vi "NIIE_KeyDown.vi"(6 "PlatMods":T9, 7 "Type":T1, 8 "Error":errorcluster, 9 "VKey":T10, 10 "Char":i16, 11 "Data":T2={"Class"={"Ants"=refnum, "Layer"=refnum, "Templates"=refnum, "Icon"=refnum, "Glyph"=refnum, "Settings"=refnum, "Tools"=refnum}, "Ref"={"Add Layer"=refnum, "Remove Layer"=refnum, "Line Text"=[], "Body Text Spec"=refnum, "DNL_Font"=refnum, "glyph path str"=refnum, "templates path str"=refnum, "Arrow Up"=refnum, "Arrow Down"=refnum, "IE VI Ref"=refnum, "Glyphs tree"=refnum, "Templates tree"=refnum, "Layer Icon Text"=refnum, "Layer Template"=refnum, "Clipboard"=refnum, "BW icon in"=refnum, "Color icon in"=refnum, "Layer Clust"=refnum, "Body Text"=refnum, "DNL_Framework Templates"=refnum, "Search Templates"=refnum, "TextMarker"=refnum, "Tab Control"=refnum, "Search Glyphs"=refnum, "Line Color"=refnum, "DNL_Glyphs []"=refnum, "Fill Color"=refnum, "Tools"=refnum, "Glyphs tree"=refnum, "Icon"=refnum, "Preview"=refnum, "Ants"=refnum, "Terminals"=refnum, "menu reference"=refnum, "LayerNames"=[], "GlyphLoadAnimation"=refnum, "TemplateLoadAnimation"=refnum, "refreshGlyphs"=refnum, "refreshTemplates"=refnum}, "Support"={"AntsRect"={"left"=0, "top"=0, "right"=0, "bottom"=0}, "Mouse Move Coords"={"Horizontal"=0, "Vertical"=0}, "Mouse Down Coords"={"Horizontal"=0, "Vertical"=0}, "Temp Coord"={"Horizontal"=0, "Vertical"=0}, "Action"=enum."Default", "Edge Color"=4914962, "Fill Color"=16860, "Mouse Down?"=FALSE, "Draft Mode?"=FALSE, "Temp Icon"=bytes[3102], "CTRL Pressed"=FALSE, "Move Selection?"=FALSE, "AntsRect Orig"={"left"=0, "top"=0, "right"=0, "bottom"=0}, "Text"="", "TM Set?"=FALSE, "Mouse inside icon?"=FALSE, "Tool (old value)"=0, "Pencil Move Color"=0, "Swap Colors?"=FALSE, "Shift pressed?"=FALSE}}) -> (0 "Error Out":errorcluster, 1 "Discard? Out":bool, 3 "Data Out":T2={"Class"={"Ants"=refnum, "Layer"=refnum, "Templates"=refnum, "Icon"=refnum, "Glyph"=refnum, "Settings"=refnum, "Tools"=refnum}, "Ref"={"Add Layer"=refnum, "Remove Layer"=refnum, "Line Text"=[], "Body Text Spec"=refnum, "DNL_Font"=refnum, "glyph path str"=refnum, "templates path str"=refnum, "Arrow Up"=refnum, "Arrow Down"=refnum, "IE VI Ref"=refnum, "Glyphs tree"=refnum, "Templates tree"=refnum, "Layer Icon Text"=refnum, "Layer Template"=refnum, "Clipboard"=refnum, "BW icon in"=refnum, "Color icon in"=refnum, "Layer Clust"=refnum, "Body Text"=refnum, "DNL_Framework Templates"=refnum, "Search Templates"=refnum, "TextMarker"=refnum, "Tab Control"=refnum, "Search Glyphs"=refnum, "Line Color"=refnum, "DNL_Glyphs []"=refnum, "Fill Color"=refnum, "Tools"=refnum, "Glyphs tree"=refnum, "Icon"=refnum, "Preview"=refnum, "Ants"=refnum, "Terminals"=refnum, "menu reference"=refnum, "LayerNames"=[], "GlyphLoadAnimation"=refnum, "TemplateLoadAnimation"=refnum, "refreshGlyphs"=refnum, "refreshTemplates"=refnum}, "Support"={"AntsRect"={"left"=0, "top"=0, "right"=0, "bottom"=0}, "Mouse Move Coords"={"Horizontal"=0, "Vertical"=0}, "Mouse Down Coords"={"Horizontal"=0, "Vertical"=0}, "Temp Coord"={"Horizontal"=0, "Vertical"=0}, "Action"=enum."Default", "Edge Color"=4914962, "Fill Color"=16860, "Mouse Down?"=FALSE, "Draft Mode?"=FALSE, "Temp Icon"=bytes[3102], "CTRL Pressed"=FALSE, "Move Selection?"=FALSE, "AntsRect Orig"={"left"=0, "top"=0, "right"=0, "bottom"=0}, "Text"="", "TM Set?"=FALSE, "Mouse inside icon?"=FALSE, "Tool (old value)"=0, "Pencil Move Color"=0, "Swap Colors?"=FALSE, "Shift pressed?"=FALSE}})   [LabVIEW 2021]
uses:
  <vilib>/event_ctls.llb/eventvkey.ctl
  Controls/IE Data.ctl
  Class/Ants/Ants.lvclass
  Class/FakedArray/FakedArray.lvclass
  Class/Icon Library/Glyph.lvclass
  Class/Settings/Settings.lvclass
  Class/Tools/Tools Paint.lvclass
  vi.lib/LabVIEW Icon API/lv_icon/Classes/Icon/Icon.lvclass
  Controls/IE Classes.ctl
  Controls/References Cluster.ctl
  Controls/SupportClass.ctl
  <vilib>/Utility/miscctls.llb/LVPoint32TypeDef.ctl
  Controls/ENUM_SupportClass_Action.ctl
  vi.lib/LabVIEW Icon API/lv_icon/Controls/IEColor.ctl
  <vilib>/event_ctls.llb/lveventtype.ctl
  vi.lib/LabVIEW Icon API/lv_icon/lv_icon.lvlib
panel:
  in  "Layer name":string="Clipboard"
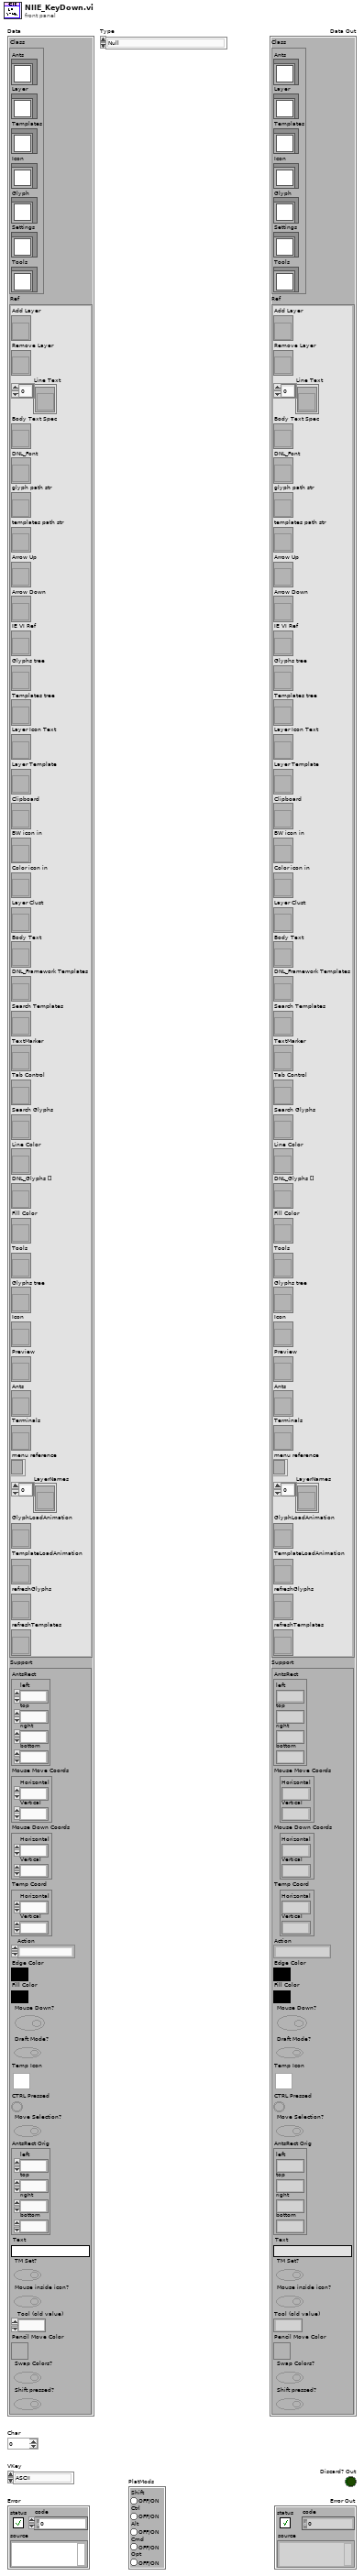
[diagram p1: front panel]
types:
  T1 = typedef "lveventtype.ctl" = enum32{"Null", "Timeout", "Annotation Menu Selection", "Annotation Menu Selection?", "App Instance Close", "App Instance Close?", "Autoscale Range Change", "Bookmark Info Change", "Cell Edit", "Cell Edit?", "Cursor Grab", "Cursor Grab?", "Cursor Menu Selection", "Cursor Menu Selection?", "Cursor Move", "Cursor Release", "Data Change", "Direction Change", "Display State Change", "Drag Ended", "Drag Enter", "Drag Leave", "Drag Over", "Drag Source Update", "Drag Starting", "Drag Starting?", "Drop", "Exec State Change", "Key Down", "Key Down?", "Key Repeat", "Key Repeat?", "Key Up", "Listbox Double Click", "Menu Activation?", "Menu Selection (App)", "Menu Selection? (App)", "Menu Selection (User)", "Mouse Down", "Mouse Down?", "Mouse Enter", "Mouse Leave", "Mouse Move", "Mouse Up", "Mouse Wheel", "NI Security User Change (App)", "Pane Size", "Panel Close", "Panel Close?", "Panel Resize", "Plot Attribute Change", "Scale Range Change", "Shortcut Menu Activation?", "Shortcut Menu Selection (App)", "Shortcut Menu Selection? (App)", "Shortcut Menu Selection (User)", "Tree Double Click", "Tree Drag", "Tree Drag?", "Tree Drop", "Tree Drop?", "Tree Item Close", "Tree Item Close?", "Tree Item Open", "Tree Item Open?", "User Event", "Value Change"}
  T2 = typedef "IE Data.ctl" = cluster{"Class":T3, "Ref":T4, "Support":T5}
  T3 = typedef "IE Classes.ctl" = cluster{"Ants":refnum<class "Ants.lvclass">, "Layer":refnum<class "FakedArray.lvclass">, "Templates":refnum<class "FakedArray.lvclass">, "Icon":refnum<class "Icon.lvclass">, "Glyph":refnum<class "Glyph.lvclass">, "Settings":refnum<class "Settings.lvclass">, "Tools":refnum<class "Tools Paint.lvclass">}
  T4 = typedef "References Cluster.ctl" = cluster{"Add Layer":refnum<vi>, "Remove Layer":refnum<vi>, "Line Text":refnum<vi>[], "Body Text Spec":refnum<vi>, "DNL_Font":refnum<vi>, "glyph path str":refnum<vi>, "templates path str":refnum<vi>, "Arrow Up":refnum<vi>, "Arrow Down":refnum<vi>, "IE VI Ref":refnum<vi>, "Glyphs tree":refnum<vi>, "Templates tree":refnum<vi>, "Layer Icon Text":refnum<vi>, "Layer Template":refnum<vi>, "Clipboard":refnum<vi>, "BW icon in":refnum<vi>, "Color icon in":refnum<vi>, "Layer Clust":refnum<vi>, "Body Text":refnum<vi>, "DNL_Framework Templates":refnum<vi>, "Search Templates":refnum<vi>, "TextMarker":refnum<vi>, "Tab Control":refnum<vi>, "Search Glyphs":refnum<vi>, "Line Color":refnum<vi>, "DNL_Glyphs []":refnum<vi>, "Fill Color":refnum<vi>, "Tools":refnum<vi>, "Glyphs tree":refnum<vi>, "Icon":refnum<vi>, "Preview":refnum<vi>, "Ants":refnum<vi>, "Terminals":refnum<vi>, "menu reference":refnum<k9>, "LayerNames":refnum<vi>[], "GlyphLoadAnimation":refnum<vi>, "TemplateLoadAnimation":refnum<vi>, "refreshGlyphs":refnum<vi>, "refreshTemplates":refnum<vi>}
  T5 = typedef "SupportClass.ctl" = cluster{"AntsRect":cluster{"left":i16, "top":i16, "right":i16, "bottom":i16}, "Mouse Move Coords":T6, "Mouse Down Coords":T6, "Temp Coord":T6, "Action":T7, "Edge Color":T8, "Fill Color":T8, "Mouse Down?":bool, "Draft Mode?":bool, "Temp Icon":picture, "CTRL Pressed":bool, "Move Selection?":bool, "AntsRect Orig":cluster{"left":i16, "top":i16, "right":i16, "bottom":i16}, "Text":string, "TM Set?":bool, "Mouse inside icon?":bool, "Tool (old value)":u32, "Pencil Move Color":u32, "Swap Colors?":bool, "Shift pressed?":bool}
  T6 = typedef "LVPoint32TypeDef.ctl" = cluster{"Horizontal":i32, "Vertical":i32}
  T7 = typedef "ENUM_SupportClass_Action.ctl" = enum16{"Default", "Move Selection", "Glyph Library", "Tool"}
  T8 = typedef "IEColor.ctl" = u32
  T9 = cluster{"Shift":bool, "Ctrl":bool, "Alt":bool, "Cmd":bool, "Opt":bool}
  T10 = typedef "eventvkey.ctl" = enum16{"ASCII", "Enter", "Return", "Shift", "Ctrl", "Alt", "Cmd", "Opt", "Caps", "NumLock", "Clear", "Break", "Up", "Down", "Left", "Right", "Insert", "Delete", "Home", "End", "PageUp", "PageDown", "Escape", "Help", "Pause", "ScrollLock", "F1", "F2", "F3", "F4", "F5", "F6", "F7", "F8", "F9", "F10", "F11", "F12", "F13", "F14", "F15", "F16", "F17", "F18", "F19", "F20", "F21", "F22", "F23", "F24", "Play", "VolumeUp", "VolumeDown", "Mute", "Two Byte Char"}
  T11 = cluster{"left":i16, "top":i16, "right":i16, "bottom":i16}
  T12 = enum32{"Pencil", "Line", "Dropper", "Fill", "Rectangle", "Filled Rectangle", "Ellipse", "Filled Ellipse", "Eraser", "Text", "Select", "Move"}
  T13 = typedef "Cluster_Path&Icon.ctl" = cluster{"Rectangle":cluster{"left":i16, "top":i16, "right":i16, "bottom":i16}, "Path":path, "Image":picture, "Filter":string, "FileName":string}
  T14 = cluster{"left":i16, "top":i16, "bottom":i16, "right":i16}
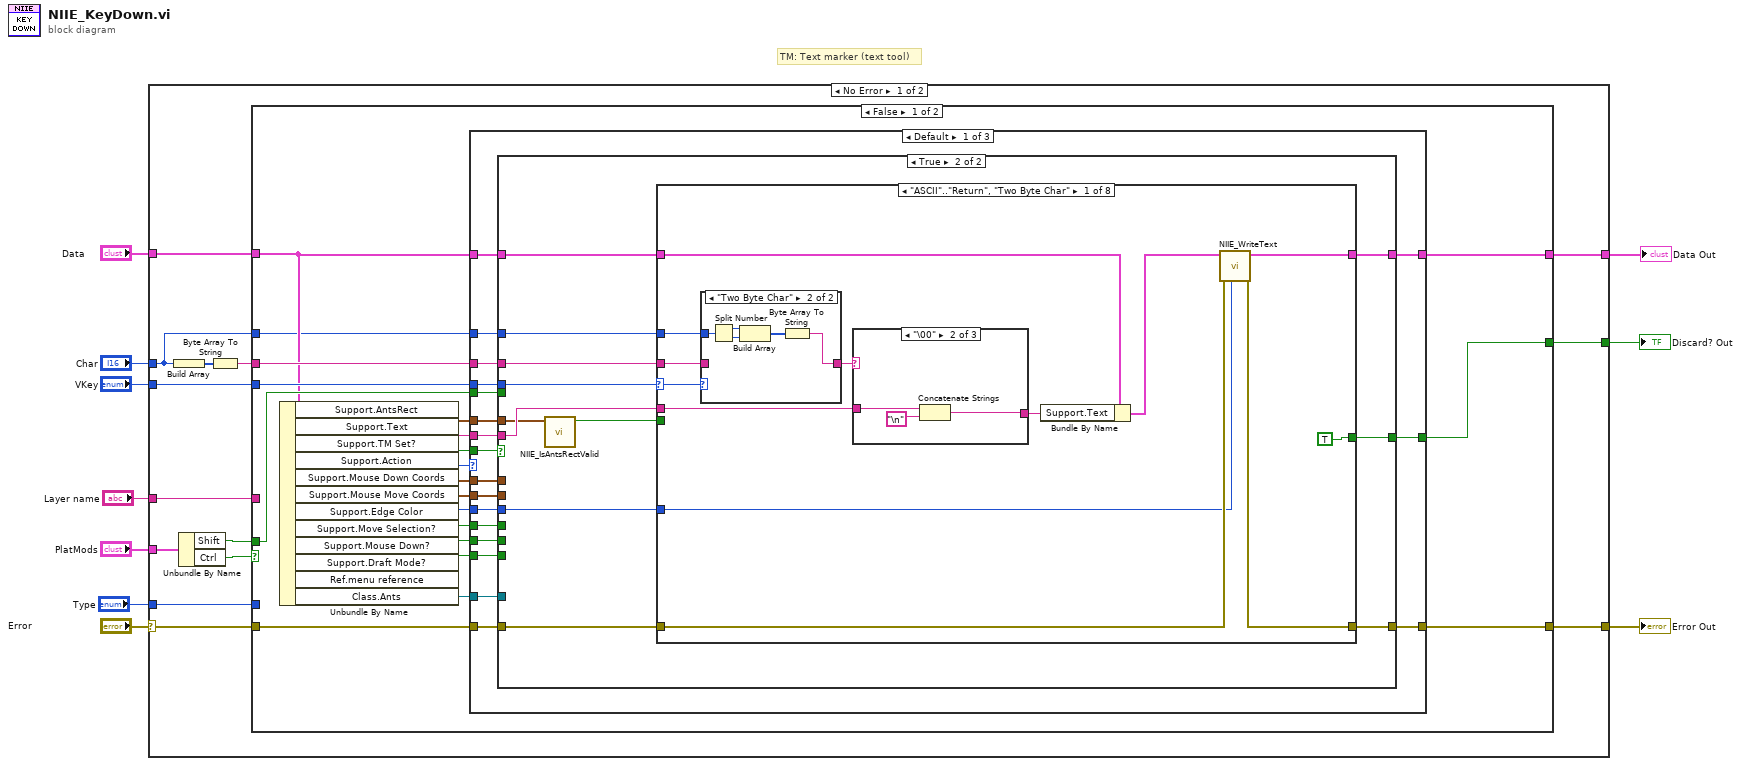
[diagram p0: block diagram]
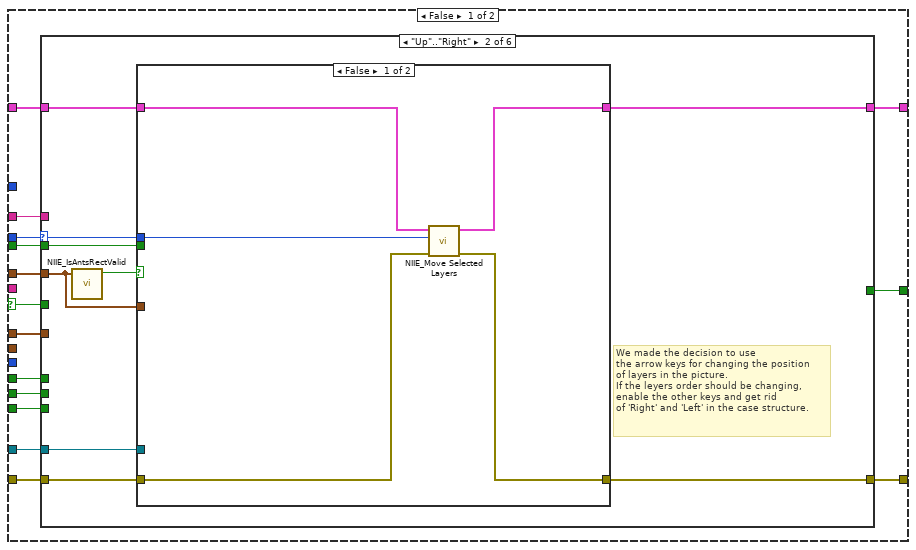
[diagram p2: hidden frame]
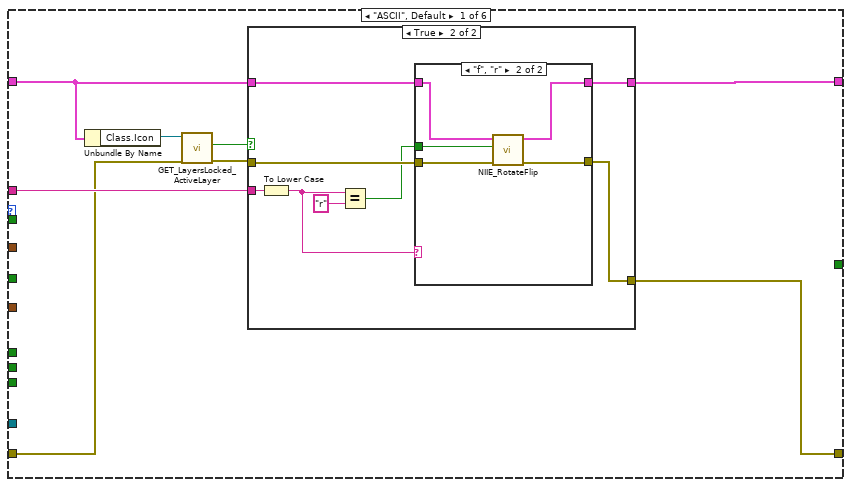
[diagram p3: hidden frame]
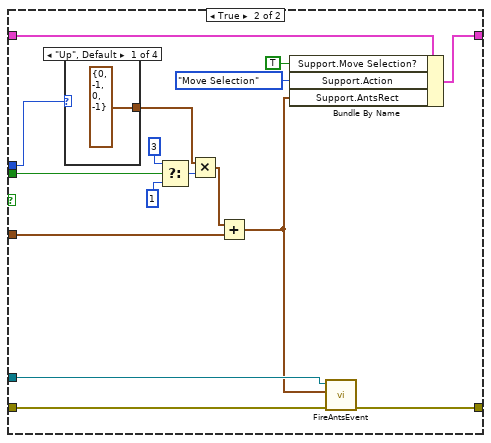
[diagram p6: hidden frame]
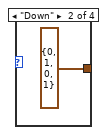
[diagram p7: hidden frame]
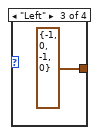
[diagram p8: hidden frame]
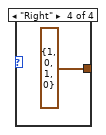
[diagram p9: hidden frame]
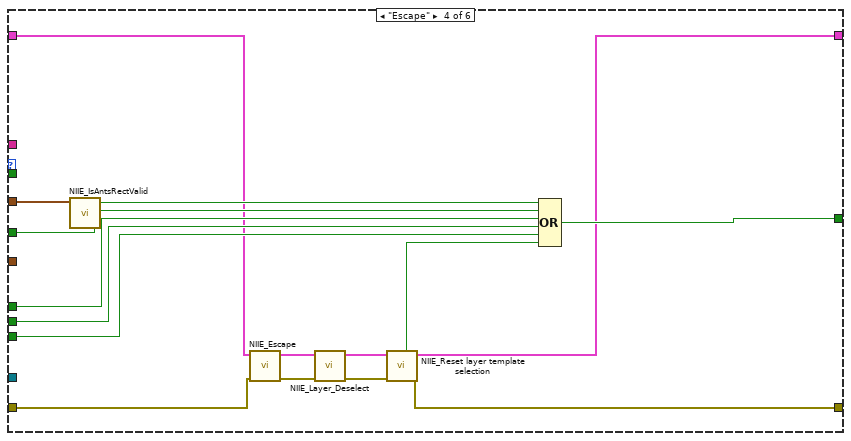
[diagram p11: hidden frame]
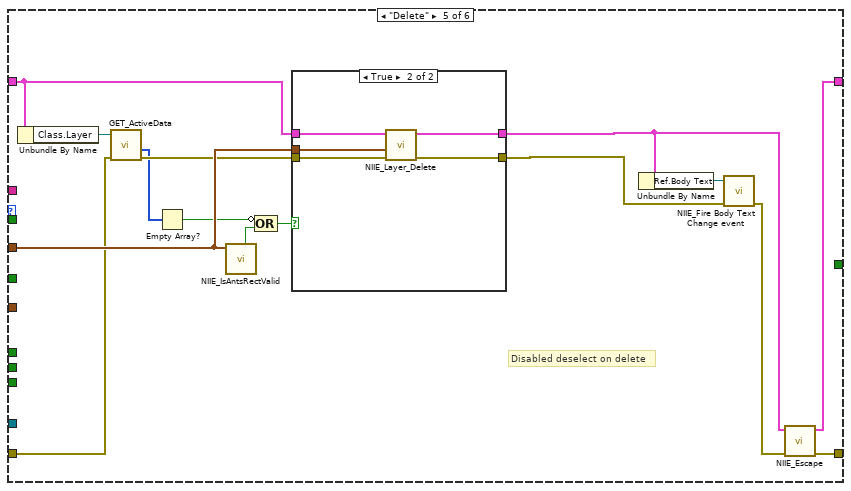
[diagram p12: hidden frame]
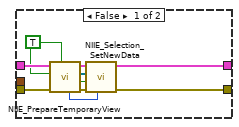
[diagram p13: hidden frame]
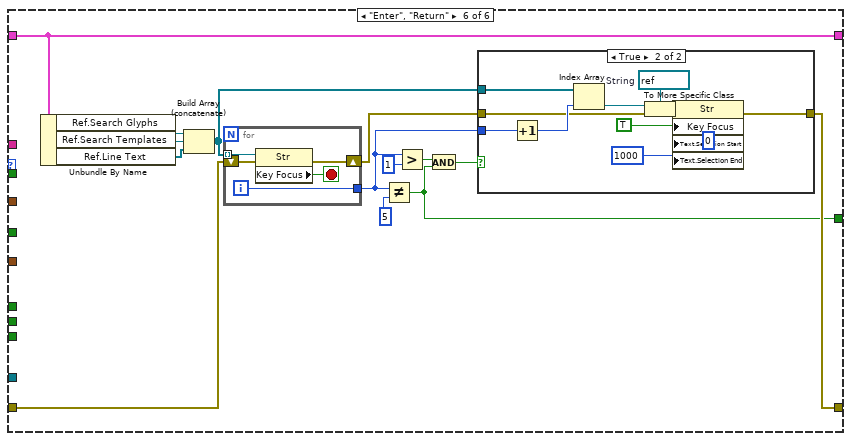
[diagram p14: hidden frame]
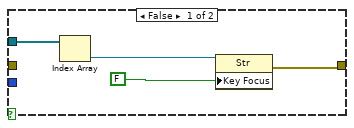
[diagram p15: hidden frame]
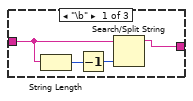
[diagram p17: hidden frame]
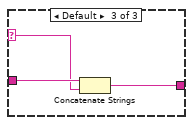
[diagram p18: hidden frame]
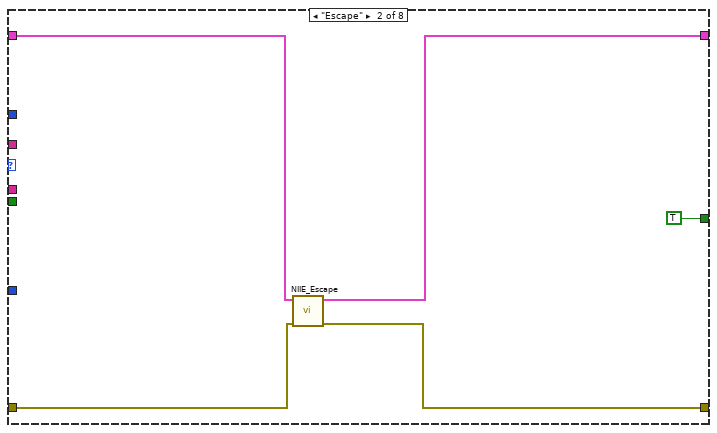
[diagram p19: hidden frame]
diagram:
  # "TM: Text marker (text tool)"
  n1 = case shown="No Error" "Error" {
    selector: "Error" -> [w17 w697]
    tunnel: [w21 w697] -> w9
    tunnel: "VKey" -> [w24 _]
    tunnel: "Char" -> [w12 _]
    tunnel: "PlatMods" -> [w20 _]
    tunnel: [w18 _] -> w5
    tunnel: "Data" -> [w15 w696]
    tunnel: [w14 w696] -> w3
    tunnel: "Type" -> [w13 _]
    tunnel: "Layer name" -> [w11 _]
    frame No Error {
      n2 = Build Array(w12) -> (w23:i16[])
      n3 = Unbundle By Name(w20) -> ("Shift"=w16:bool, "Ctrl"=w19:bool)
      n4 = Byte Array To String(unsigned byte array=w23) -> (string=w22:string)
      n5 = case shown="False" w19 {
        selector: w19 -> [_ w484]
        tunnel: w24 -> [w44 _]
        tunnel: w22 -> [w43 w482]
        tunnel: [w28 w494] -> w21
        tunnel: [w32 w481] -> w18
        tunnel: w17 -> [w30 w497]
        tunnel: w16 -> [w31 w485]
        tunnel: w15 -> [w29 w496]
        tunnel: [w26 w495] -> w14
        tunnel: w13 -> [_ w489]
        tunnel: w12 -> [w25 _]
        tunnel: w11 -> [_ w479]
        frame False {
          n6 = Unbundle By Name(w29) -> ("Support.AntsRect"=w37:T11, "Support.Text"=w40:string, "Support.TM Set?"=w41:bool, "Support.Action"=w42:T7, "Support.Mouse Down Coords"=w39:T6, "Support.Mouse Move Coords"=w36:T6, "Support.Edge Color"=w38:T8, "Support.Move Selection?"=w35:bool, "Support.Mouse Down?"=w34:bool, "Support.Draft Mode?"=w33:bool, "Class.Ants"=w27:refnum<class "Ants.lvclass">)  [unwired: 1 out]
          n7 = case shown="Default" w42 {
            tunnel: w44 -> [w63 w329 w396]
            tunnel: w43 -> [w58 w328 _]
            tunnel: w30 -> [w61 w327 w398]
            tunnel: [w62 w326 w397] -> w28
            tunnel: w41 -> [w60 w324 w394]
            tunnel: w40 -> [w59 _ _]
            tunnel: w39 -> [w57 _ _]
            tunnel: w38 -> [w56 _ _]
            tunnel: w37 -> [w55 w325 w395]
            tunnel: w36 -> [w54 w317 _]
            tunnel: w35 -> [w53 w323 w393]
            tunnel: w34 -> [w52 w322 w392]
            tunnel: w33 -> [w51 w321 w391]
            tunnel: [w50 w320 w390] -> w32
            tunnel: w31 -> [w49 _ w386]
            tunnel: w29 -> [w48 w319 w389]
            tunnel: [w47 w318 w388] -> w26
            tunnel: w27 -> [w45 _ w387]
            tunnel: w25 -> [w46 _ _]
            frame Default {
              n8 = case shown="True" w60 {
                selector: w60 -> [w69 _]
                tunnel: w63 -> [w77 w231]
                tunnel: [w76 w230] -> w62
                tunnel: w61 -> [w78 w229]
                tunnel: w59 -> [_ w228]
                tunnel: w58 -> [w75 w227]
                tunnel: w57 -> [w73 _]
                tunnel: w56 -> [_ w224]
                tunnel: w55 -> [w74 w226]
                tunnel: w54 -> [_ _]
                tunnel: w53 -> [w72 _]
                tunnel: w52 -> [w71 _]
                tunnel: w51 -> [w70 _]
                tunnel: [w68 w223] -> w50
                tunnel: w49 -> [w67 _]
                tunnel: w48 -> [w66 w222]
                tunnel: [w65 w221] -> w47
                tunnel: w46 -> [_ w220]
                tunnel: w45 -> [w64 _]
                frame False {
                  n9 = case shown="\"Up\"..\"Right\"" w77 {
                    selector: w77 -> [_ w110 _ _ _ _]
                    tunnel: w78 -> [w82 w112 w139 w155 w163 w198]
                    tunnel: [w85 w111 w139 w152 w170 w195] -> w76
                    tunnel: w75 -> [w86 _ _ _ _ _]
                    tunnel: w74 -> [_ w105 _ w150 w167 _]
                    tunnel: w73 -> [_ _ _ _ _ _]
                    tunnel: w72 -> [_ _ _ w148 _ _]
                    tunnel: w71 -> [_ _ _ w147 _ _]
                    tunnel: w70 -> [_ _ _ w146 _ _]
                    tunnel: w69 -> [_ _ _ w149 _ _]
                    tunnel: [_ _ _ w145 _ w187] -> w68
                    tunnel: w67 -> [_ w109 _ _ _ _]
                    tunnel: w66 -> [w84 w108 w138 w143 w164 w199]
                    tunnel: [w83 w107 w138 w140 w169 w199] -> w65
                    tunnel: w64 -> [_ w104 _ _ _ _]
                    frame "ASCII", Default {
                      n10 = Unbundle By Name(w84) -> ("Class.Icon"=w80:refnum<class "Icon.lvclass">)
                      n11 = call-dynamic "GET_LayersLocked_ActiveLayer.vi"("error in (no error)"=w82, "Icon.lvclass in"=w80) -> ("error out"=w81:errorcluster, "Layers Locked?"=w79:bool)  [unwired: 8 out]
                      n12 = case shown="True" w79 {
                        tunnel: w86 -> [_ w93]
                        tunnel: w81 -> [w88 w96]
                        tunnel: [w88 w95] -> w85
                        tunnel: w84 -> [w87 w90]
                        tunnel: [w87 w89] -> w83
                        frame False {
                        }
                        frame True {
                          n13 = To Lower Case(string=w93) -> (all lower case string=w91:string)
                          n14 = Equal?(x=w91, y="r") -> (x = y?=w92:bool)
                          n15 = case shown="\"f\", \"r\"" w91 {
                            tunnel: w96 -> [w98 w103]
                            tunnel: [w98 w101] -> w95
                            tunnel: w92 -> [_ w102]
                            tunnel: w90 -> [w97 w100]
                            tunnel: [w97 w99] -> w89
                            frame Default {
                            }
                            frame "f", "r" {
                              n16 = call "NIIE_RotateFlip.vi"("Error"=w103, "Rotate"=w102, "Data"=w100) -> ("Error Out"=w101:errorcluster, "Data Out"=w99:T2)  [unwired: 3 in, 4 out]
                            }
                          }
                        }
                      }
                    }
                    frame "Up".."Right" {
                      # "We made the decision to use\nthe arrow keys for changing the position\nof layers in the picture.\nIf the leyers order should be changing,\nenable the other keys and get rid\nof 'Right' and 'Left' in the case structure."
                      n17 = call "NIIE_IsAntsRectValid.vi"("Image Range"=w105) -> ("Valid? Out"=w106:bool)  [unwired: 10 out]
                      n18 = case shown="False" w106 {
                        tunnel: w112 -> [w117 w121]
                        tunnel: [w116 w120] -> w111
                        tunnel: w110 -> [w115 w124]
                        tunnel: w109 -> [_ w123]
                        tunnel: w108 -> [w114 w133]
                        tunnel: [w113 w131] -> w107
                        tunnel: w105 -> [_ w122]
                        tunnel: w104 -> [_ w119]
                        frame False {
                          n19 = call "NIIE_Move Selected Layers.vi"("Error"=w117, "VKey"=w115, "Data"=w114) -> ("Error Out"=w116:errorcluster, "Data Out"=w113:T2)  [unwired: 1 in, 6 out]
                        }
                        frame True {
                          n20 = case shown="\"Up\", Default" w124 {
                            tunnel: [T11 {"left"=0, "top"=-1, "right"=0, "bottom"=-1} ("y") T11 {"left"=0, "top"=1, "right"=0, "bottom"=1} ("y") T11 {"left"=-1, "top"=0, "right"=-1, "bottom"=0} ("y") T11 {"left"=1, "top"=0, "right"=1, "bottom"=0} ("y")] -> w129
                            frame "Up", Default {
                            }
                            frame "Down" {
                            }
                            frame "Left" {
                            }
                            frame "Right" {
                            }
                          }
                          n21 = Select(t=i16 3 ("left"), s=w123, f=i16 1 ("left")) -> (s? t:f=w126:i16)
                          n22 = Multiply(x=w129, y=w126) -> (x*y=w125:T11)
                          n23 = Add(x=w125, y=w122) -> (x+y=w118:T11)
                          n24 = Bundle By Name(cluster=w133, "Support.Move Selection?"=TRUE, "Support.Action"=ENUM_SupportClass_Action."Move Selection", "Support.AntsRect"=w118) -> (w131:T2)
                          n25 = call "FireAntsEvent.vi"("error in (no error)"=w121, "Rectangle (default: deselect)"=w118, "Ants in"=w119) -> ("error out"=w120:errorcluster)  [unwired: 1 in, 7 out]
                        }
                      }
                    }
                    frame "Shift" {
                    }
                    frame "Escape" {
                      n26 = call "NIIE_IsAntsRectValid.vi"("Image Range"=w150) -> ("Valid? Out"=w151:bool)  [unwired: 10 out]
                      n27 = call "NIIE_Escape.vi"("Error"=w155, "Data"=w143) -> ("Error Out"=w154:errorcluster, "Data Out"=w142:T2)  [unwired: 8 out]
                      n28 = call "NIIE_Layer_Deselect.vi"("Error"=w154, "Data"=w142) -> ("Error Out"=w153:errorcluster, "Data Out"=w141:T2)  [unwired: 8 out]
                      n29 = call "NIIE_Reset layer template selection.vi"("Error"=w153, "Data"=w141) -> ("Error Out"=w152:errorcluster, "Data Out"=w140:T2, "Layers Selected? Out"=w144:bool)  [unwired: 1 in, 6 out]
                      n30 = Compound Arithmetic op=OR(w151, w149, w148, w147, w146, w144) -> (w145:bool)
                    }
                    frame "Delete" {
                      # "Disabled deselect on delete"
                      n31 = Unbundle By Name(w164) -> ("Class.Layer"=w165:refnum<class "FakedArray.lvclass">)
                      n32 = call-dynamic "GET_ActiveData.vi"("Error"=w163, "FakedArray"=w165) -> ("Error Out"=w162:errorcluster, "Active Data [] Out"=w161:i32[])  [unwired: 4 in, 4 out]
                      n33 = Empty Array?(array=w161) -> (empty?=w159:bool)
                      n34 = call "NIIE_IsAntsRectValid.vi"("Image Range"=w167) -> ("Max. Rect Size? Out"=w160:bool)  [unwired: 10 out]
                      n35 = Compound Arithmetic op=OR(invert w159, w160) -> (w158:bool)
                      n36 = case shown="True" w158 {
                        tunnel: w164 -> [w180 w185]
                        tunnel: [w179 w183] -> w168
                        tunnel: [w178 w184] -> w157
                        tunnel: w162 -> [w171 w182]
                        tunnel: w167 -> [_ w181]
                        frame False {
                          w177 = TRUE ("Delete Selected Area?")
                          n37 = call "NIIE_PrepareTemporaryView.vi"("Delete Selected Area?"=w177, "Error"=w171, "Valid Selection?"=w177, "Data"=w180) -> ("Error Out"=w174:errorcluster, "Highlighted? Out"=w175:bool, "All Layers Out"=w176:refnum<class "Layer.lvclass">[], "Data Out"=w172:T2, "#Active Layer Out"=w173:i32)  [unwired: 1 in, 2 out]
                          n38 = call "NIIE_Selection_SetNewData.vi"("#Active Layer"=w173, "Error"=w174, "Highlighted?"=w175, "All Layers"=w176, "Data"=w172) -> ("Error Out"=w179:errorcluster, "Data Out"=w178:T2)  [unwired: 1 in, 3 out]
                        }
                        frame True {
                          n39 = call "NIIE_Layer_Delete.vi"("Error"=w182, "AntsRect"=w181, "Data"=w185) -> ("Error Out"=w183:errorcluster, "Data Out"=w184:T2)  [unwired: 5 out]
                        }
                      }
                      n40 = Unbundle By Name(w157) -> ("Ref.Body Text"=w156:refnum<vi>)
                      n41 = call "NIIE_Fire Body Text Change event.vi"("error in"=w168, "Ref.Body Text"=w156) -> ("error out"=w166:errorcluster)  [unwired: 2 in, 7 out]
                      n42 = call "NIIE_Escape.vi"("Error"=w166, "Data"=w157) -> ("Error Out"=w170:errorcluster, "Data Out"=w169:T2)  [unwired: 8 out]
                    }
                    frame "Enter", "Return" {
                      n43 = Unbundle By Name(w199) -> ("Ref.Search Glyphs"=w191:refnum<vi>, "Ref.Search Templates"=w192:refnum<vi>, "Ref.Line Text"=w194:refnum<vi>[])
                      n44 = Build Array (concatenate)(w191, w192, w194) -> (w193:refnum<vi>[])
                      n45 = for {
                        tunnel: w193 -> [w219] mode=indexing
                        shift-right: [w218] -> w196
                        shift-left: w198 -> [w217]
                        tunnel: [w216] -> w190
                        i -> [w216]
                        stop <- w215 stop-if-true
                        n46 = property class="Str"(reference=w219, error in=w217) -> (error out=w218:errorcluster, "Key Focus"=w215:bool)  [unwired: 1 out]
                      }
                      n47 = Not Equal?(x=w190, y=5) -> (x != y?=w187:bool)
                      n48 = Greater?(x=w190, y=1) -> (0:w188:bool)
                      n49 = And(x=w188, y=w187) -> (x .and. y?=w186:bool)
                      n50 = case shown="True" w186 {
                        tunnel: w190 -> [_ w213]
                        tunnel: w193 -> [w203 w214]
                        tunnel: w196 -> [_ w210]
                        tunnel: [w200 w208] -> w195
                        frame False {
                          n51 = Index Array(array=w203) -> (element=w202:refnum<vi>)  [unwired: 1 in]
                          n52 = property class="Str"(reference=w202, "Key Focus"=FALSE) -> (error out=w200:errorcluster)  [unwired: 1 in, 1 out]
                        }
                        frame True {
                          w204 = refnum<vi> refnum  # String
                          n53 = Increment(x=w213) -> (x+1=w212:i32)
                          n54 = Index Array(array=w214, index=w212) -> (element=w211:refnum<vi>)
                          n55 = To More Specific Class(target class=w204, reference=w211) -> (specific class reference=w205:refnum<vi>)  [unwired: 1 in, 1 out]
                          n56 = property class="Str"(reference=w205, error in=w210, "Key Focus"=TRUE, "Text.Selection Start"=u32 0 ("Text.Selection:Start"), "Text.Selection End"=u32 1000 ("Text.Selection:End")) -> (error out=w208:errorcluster)  [unwired: 1 out]
                        }
                      }
                    }
                  }
                }
                frame True {
                  n57 = call "NIIE_IsAntsRectValid.vi"("Image Range"=w226) -> ("Valid? Out"=w225:bool)  [unwired: 10 out]
                  n58 = case shown="\"ASCII\"..\"Return\", \"Two Byte Char\"" w231 {
                    selector: w231 -> [w235 _ _ _ _ _ _ _]
                    tunnel: [w242 w264 w267 w271 w296 w302 w308 w314] -> w230
                    tunnel: w229 -> [w243 w265 w267 w272 w297 w303 w309 w315]
                    tunnel: w228 -> [w244 _ _ w273 _ _ _ _]
                    tunnel: w227 -> [w233 _ _ _ _ _ _ _]
                    tunnel: w224 -> [w241 _ _ _ w298 w304 w310 w316]
                    tunnel: w225 -> [_ _ _ w270 _ _ _ _]
                    tunnel: [TRUE TRUE _ _ _ _ _ _] -> w223
                    tunnel: w222 -> [w236 w262 w266 w269 w295 w300 w307 w313]
                    tunnel: [w239 w261 w266 w268 w293 w299 w306 w311] -> w221
                    tunnel: w220 -> [w232 _ _ _ _ _ _ _]
                    frame "ASCII".."Return", "Two Byte Char" {
                      n59 = case shown="\"Two Byte Char\"" w235 {
                        tunnel: [w245 w246] -> w234
                        tunnel: w233 -> [w245 _]
                        tunnel: w232 -> [_ w250]
                        frame "ASCII", Default {
                        }
                        frame "Two Byte Char" {
                          n60 = Split Number(x=w250) -> (hi(x)=w248:u8, lo(x)=w249:u8)
                          n61 = Build Array(w248, w249) -> (w247:u8[])
                          n62 = Byte Array To String(unsigned byte array=w247) -> (string=w246:string)
                        }
                      }
                      n63 = case shown="\"\\00\"" w234 {
                        selector: w234 -> [_ _ w258]
                        tunnel: w244 -> [w252 w257 w260]
                        tunnel: [w251 w256 w259] -> w238
                        frame "\b" {
                          n64 = String Length(string=w252) -> (length=w254:i32)
                          n65 = Decrement(x=w254) -> (x-1=w253:i32)
                          n66 = Search/Split String(string=w252, offset (0)=w253) -> (substring before match=w251:string)  [unwired: 3 out]
                        }
                        frame "\u0000\u0000" {
                          n67 = Concatenate Strings(w257, "\n") -> (w256:string)
                        }
                        frame Default {
                          n68 = Concatenate Strings(w260, w258) -> (w259:string)
                        }
                      }
                      n69 = Bundle By Name(cluster=w236, "Support.Text"=w238) -> (w237:T2)
                      n70 = call "NIIE_WriteText.vi"("Text Color"=w241, "Error"=w243, "Data"=w237) -> ("Error Out"=w242:errorcluster, "Data Out"=w239:T2)  [unwired: 2 in, 5 out]
                    }
                    frame "Escape" {
                      n71 = call "NIIE_Escape.vi"("Error"=w265, "Data"=w262) -> ("Error Out"=w264:errorcluster, "Data Out"=w261:T2)  [unwired: 8 out]
                    }
                    frame Default {
                    }
                    frame "Delete" {
                      n72 = case shown="True" w270 {
                        tunnel: w273 -> [_ _]
                        tunnel: w272 -> [w275 w284]
                        tunnel: [w275 w287] -> w271
                        tunnel: w269 -> [w274 w277]
                        tunnel: [w274 w281] -> w268
                        frame False {
                        }
                        frame True {
                          w292 = TRUE ("Delete Selected Area?")
                          n73 = Unbundle By Name(w277) -> ("Ref.Body Text"=w276:refnum<vi>)
                          n74 = call "NIIE_Fire Body Text Change event.vi"("error in"=w284, "Ref.Body Text"=w276) -> ("error out"=w285:errorcluster)  [unwired: 2 in, 7 out]
                          n75 = call "NIIE_PrepareTemporaryView.vi"("Delete Selected Area?"=w292, "Error"=w285, "Valid Selection?"=w292, "Data"=w277) -> ("Error Out"=w288:errorcluster, "Highlighted? Out"=w290:bool, "All Layers Out"=w291:refnum<class "Layer.lvclass">[], "Data Out"=w283:T2, "#Active Layer Out"=w289:i32)  [unwired: 1 in, 2 out]
                          n76 = call "NIIE_Selection_SetNewData.vi"("#Active Layer"=w289, "Error"=w288, "Highlighted?"=w290, "All Layers"=w291, "Data"=w283) -> ("Error Out"=w286:errorcluster, "Data Out"=w282:T2)  [unwired: 1 in, 3 out]
                          n77 = call "NIIE_Layer_View.vi"("Add To Undo?"=TRUE ("Add to Undo?"), "Error"=w286, "Data"=w282) -> ("Error Out"=w280:errorcluster, "Data Out"=w279:T2)  [unwired: 2 in, 5 out]
                          n78 = call "NIIE_Escape.vi"("Error"=w280, "Data"=w279) -> ("Error Out"=w287:errorcluster, "Data Out"=w281:T2)  [unwired: 8 out]
                        }
                      }
                    }
                    frame "Up" {
                      n79 = call "NIIE_WriteText.vi"("Text Color"=w298, "Error"=w297, "Offset"=T6 {"Horizontal"=0, "Vertical"=-1} ("y"), "Data"=w295) -> ("Error Out"=w296:errorcluster, "Data Out"=w293:T2)  [unwired: 1 in, 5 out]
                    }
                    frame "Down" {
                      n80 = call "NIIE_WriteText.vi"("Text Color"=w304, "Error"=w303, "Offset"=T6 {"Horizontal"=0, "Vertical"=1} ("y"), "Data"=w300) -> ("Error Out"=w302:errorcluster, "Data Out"=w299:T2)  [unwired: 1 in, 5 out]
                    }
                    frame "Left" {
                      n81 = call "NIIE_WriteText.vi"("Text Color"=w310, "Error"=w309, "Offset"=T6 {"Horizontal"=-1, "Vertical"=0} ("y"), "Data"=w307) -> ("Error Out"=w308:errorcluster, "Data Out"=w306:T2)  [unwired: 6 out]
                    }
                    frame "Right" {
                      n82 = call "NIIE_WriteText.vi"("Text Color"=w316, "Error"=w315, "Offset"=T6 {"Horizontal"=1, "Vertical"=0} ("y"), "Data"=w313) -> ("Error Out"=w314:errorcluster, "Data Out"=w311:T2)  [unwired: 6 out]
                    }
                  }
                }
              }
            }
            frame "Glyph Library" {
              n83 = case shown="\"ASCII\", Default" w329 {
                tunnel: w327 -> [w334 w381 w384]
                tunnel: [w333 w380 w384] -> w326
                tunnel: w328 -> [w335 _ _]
                tunnel: w325 -> [_ w378 _]
                tunnel: w324 -> [_ w377 _]
                tunnel: w323 -> [_ w376 _]
                tunnel: w322 -> [_ w375 _]
                tunnel: w321 -> [_ w374 _]
                tunnel: [_ w373 _] -> w320
                tunnel: w319 -> [w332 w372 w383]
                tunnel: [w331 w370 w382] -> w318
                tunnel: w317 -> [w330 _ _]
                frame "ASCII", Default {
                  n84 = case shown="\"F\", \"R\", \"f\", \"r\"" w335 {
                    selector: w335 -> [_ w354]
                    tunnel: w334 -> [w337 w340]
                    tunnel: [w337 w339] -> w333
                    tunnel: w332 -> [w336 w344]
                    tunnel: [w336 w341] -> w331
                    tunnel: w330 -> [_ w338]
                    frame Default {
                    }
                    frame "F", "R", "f", "r" {
                      n85 = Unbundle By Name(w344) -> ("Class.Glyph"=w345:refnum<class "Glyph.lvclass">)
                      n86 = call-dynamic "GET_ActiveGlyph.vi"("Error"=w340, "Glyph.lvclass"=w345) -> ("Error Out"=w357:errorcluster, "Path And Icon Out"=w359:T13, "Glyph.lvclass Out"=w358:refnum<class "Glyph.lvclass">)  [unwired: 7 out]
                      n87 = Unbundle By Name(w359) -> ("Image"=w361:picture, "Rectangle"=w360:T11)
                      n88 = Equal?(x=w354, y="r") -> (x = y?=w351:bool)
                      n89 = Equal?(x=w354, y="R") -> (x = y?=w352:bool)
                      n90 = Or(x=w351, y=w352) -> (x .or. y?=w346:bool)
                      n91 = call "Rotate Flip Image.vi"("Rotate?"=w346, "rect"=w360, "Temp Icon In"=w361) -> ("rect out"=w349:T14, "Temp Icon Out"=w350:picture)  [unwired: 7 out]
                      n92 = case shown="False" w346 {
                        tunnel: w350 -> [w366 w368]
                        tunnel: w349 -> [w365 w367]
                        tunnel: [w364 w368] -> w348
                        tunnel: [w363 w367] -> w347
                        frame False {
                          n93 = call "Rotate Flip Image.vi"("Rotate?"=TRUE, "rect"=w365, "Temp Icon In"=w366) -> ("rect out"=w363:T14, "Temp Icon Out"=w364:picture)  [unwired: 7 out]
                        }
                        frame True {
                        }
                      }
                      n94 = Bundle By Name(cluster=w359, "Image"=w348, "Rectangle"=w347) -> (w356:T13)
                      n95 = call "NIIE_TemporaryGlyphView.vi"("Mouse Coords Pic"=w338, "Path And Icon"=w356) -> ("Icon Out"=w342:picture)  [unwired: 9 out]
                      n96 = call-dynamic "SET_ActiveGlyph.vi"("Error"=w357, "Active Glyph"=w356, "Glyph"=w358) -> ("Error Out"=w339:errorcluster, "Glyph Out"=w343:refnum<class "Glyph.lvclass">)  [unwired: 7 out]
                      n97 = Bundle By Name(cluster=w344, "Class.Glyph"=w343, "Support.Temp Icon"=w342) -> (w341:T2)
                    }
                  }
                }
                frame "Escape" {
                  n98 = call "NIIE_IsAntsRectValid.vi"("Image Range"=w378) -> ("Valid? Out"=w379:bool)  [unwired: 10 out]
                  n99 = Compound Arithmetic op=OR(w379, w377, w376, w375, w374) -> (w373:bool)
                  n100 = call "NIIE_Escape.vi"("Error"=w381, "Data"=w372) -> ("Error Out"=w369:errorcluster, "Data Out"=w371:T2)  [unwired: 8 out]
                  n101 = call "NIIE_Reset layer template selection.vi"("Error"=w369, "Data"=w371) -> ("Error Out"=w380:errorcluster, "Data Out"=w370:T2)  [unwired: 1 in, 7 out]
                }
                frame "Ctrl" {
                  n102 = Bundle By Name(cluster=w383, "Support.CTRL Pressed"=TRUE ("CTRL Pressed")) -> (w382:T2)
                }
              }
            }
            frame "Move Selection" {
              n103 = case shown="\"Delete\"" w396 {
                selector: w396 -> [_ w405 _ _]
                tunnel: w398 -> [w400 w403 w437 w448]
                tunnel: [w400 w402 w430 w454] -> w397
                tunnel: w395 -> [_ w407 w444 w447]
                tunnel: w394 -> [_ _ w442 _]
                tunnel: w393 -> [_ _ w441 _]
                tunnel: w392 -> [_ _ w440 _]
                tunnel: w391 -> [_ _ w439 _]
                tunnel: [_ _ w438 _] -> w390
                tunnel: w389 -> [w399 w409 w434 w449]
                tunnel: [w399 w406 w431 w453] -> w388
                tunnel: w387 -> [_ w401 w436 _]
                tunnel: w386 -> [_ w404 _ _]
                frame "ASCII", Default {
                }
                frame "Up".."Right" {
                  n104 = call "NIIE_IsAntsRectValid.vi"("Image Range"=w407) -> ("Valid? Out"=w408:bool)  [unwired: 10 out]
                  n105 = case shown="True" w408 {
                    tunnel: w409 -> [w411 w425]
                    tunnel: w407 -> [_ w423]
                    tunnel: [w411 w424] -> w406
                    tunnel: w405 -> [_ w416]
                    tunnel: w404 -> [_ w421]
                    tunnel: w403 -> [w410 w415]
                    tunnel: [w410 w414] -> w402
                    tunnel: w401 -> [_ w413]
                    frame False {
                    }
                    frame True {
                      n106 = case shown="\"Up\", Default" w416 {
                        tunnel: [T11 {"left"=0, "top"=-1, "right"=0, "bottom"=-1} ("y") T11 {"left"=0, "top"=1, "right"=0, "bottom"=1} ("y") T11 {"left"=-1, "top"=0, "right"=-1, "bottom"=0} ("y") T11 {"left"=1, "top"=0, "right"=1, "bottom"=0} ("y")] -> w422
                        frame "Up", Default {
                        }
                        frame "Down" {
                        }
                        frame "Left" {
                        }
                        frame "Right" {
                        }
                      }
                      n107 = Select(t=i16 3 ("left"), s=w421, f=i16 1 ("left")) -> (s? t:f=w418:i16)
                      n108 = Multiply(x=w422, y=w418) -> (x*y=w417:T11)
                      n109 = Add(x=w417, y=w423) -> (x+y=w412:T11)
                      n110 = Bundle By Name(cluster=w425, "Support.AntsRect"=w412) -> (w424:T2)
                      n111 = call "FireAntsEvent.vi"("error in (no error)"=w415, "Rectangle (default: deselect)"=w412, "Ants in"=w413) -> ("error out"=w414:errorcluster)  [unwired: 1 in, 7 out]
                    }
                  }
                }
                frame "Escape" {
                  n112 = call "NIIE_IsAntsRectValid.vi"("Image Range"=w444) -> ("Valid? Out"=w443:bool)  [unwired: 10 out]
                  n113 = Compound Arithmetic op=OR(w443, w442, w441, w440, w439) -> (w438:bool)
                  n114 = call "FireAntsEvent.vi"("error in (no error)"=w437, "Ants in"=w436) -> ("error out"=w435:errorcluster)  [unwired: 2 in, 7 out]
                  n115 = call "NIIE_Reset layer template selection.vi"("Error"=w435, "Data"=w434) -> ("Error Out"=w433:errorcluster, "Data Out"=w432:T2)  [unwired: 1 in, 7 out]
                  n116 = call "NIIE_Escape.vi"("Error"=w433, "Data"=w432) -> ("Error Out"=w430:errorcluster, "Data Out"=w431:T2)  [unwired: 8 out]
                }
                frame "Delete" {
                  # "Disable deselect on delete"
                  n117 = call "NIIE_IsAntsRectValid.vi"("Image Range"=w447) -> ("Max. Rect Size? Out"=w450:bool)  [unwired: 10 out]
                  n118 = case shown="True" w450 {
                    tunnel: w449 -> [w464 w468]
                    tunnel: [w463 w475] -> w452
                    tunnel: [w462 w476] -> w446
                    tunnel: w448 -> [w455 w466]
                    tunnel: w447 -> [_ w474]
                    frame False {
                      w461 = TRUE ("Delete Selected Area?")
                      n119 = call "NIIE_PrepareTemporaryView.vi"("Delete Selected Area?"=w461, "Error"=w455, "Valid Selection?"=w461, "Data"=w464) -> ("Error Out"=w458:errorcluster, "Highlighted? Out"=w459:bool, "All Layers Out"=w460:refnum<class "Layer.lvclass">[], "Data Out"=w456:T2, "#Active Layer Out"=w457:i32)  [unwired: 1 in, 2 out]
                      n120 = call "NIIE_Selection_SetNewData.vi"("#Active Layer"=w457, "Error"=w458, "Highlighted?"=w459, "All Layers"=w460, "Data"=w456) -> ("Error Out"=w463:errorcluster, "Data Out"=w462:T2)  [unwired: 1 in, 3 out]
                    }
                    frame True {
                      n121 = Unbundle By Name(w468) -> ("Class.Icon"=w473:refnum<class "Icon.lvclass">)
                      n122 = call-dynamic "GET_All User Layers.vi"("error in (no error)"=w466, "Icon.lvclass in"=w473) -> ("error out"=w472:errorcluster, "User Layer"=w469:refnum<class "Layer.lvclass">[])  [unwired: 7 in, 1 out]
                      n123 = Array Size(array=w469) -> (size(s)=w470:i32)
                      n124 = for {
                        N: w470 -> [_]
                        tunnel: [w477] -> w471 mode=indexing
                        i -> [w477]
                      }
                      n125 = call "NIIE_Set active Layer programmatically.vi"("Error"=w472, "Active Layer []"=w471, "Data"=w468) -> ("Error Out"=w465:errorcluster, "Data Out"=w467:T2)  [unwired: 7 in]
                      n126 = call "NIIE_Layer_Delete.vi"("Error"=w465, "AntsRect"=w474, "Data"=w467) -> ("Error Out"=w475:errorcluster, "Data Out"=w476:T2)  [unwired: 5 out]
                    }
                  }
                  n127 = Unbundle By Name(w446) -> ("Ref.Body Text"=w445:refnum<vi>)
                  n128 = call "NIIE_Fire Body Text Change event.vi"("error in"=w452, "Ref.Body Text"=w445) -> ("error out"=w451:errorcluster)  [unwired: 2 in, 7 out]
                  n129 = call "NIIE_Escape.vi"("Error"=w451, "Data"=w446) -> ("Error Out"=w454:errorcluster, "Data Out"=w453:T2)  [unwired: 8 out]
                }
              }
            }
          }
        }
        frame True {
          n130 = Unbundle By Name(w496) -> ("Support.AntsRect"=w478:T11, "Support.Action"=w483:T7, "Support.Mouse Down?"=w492:bool, "Support.Mouse inside icon?"=w493:bool, "Ref.Tools"=w498:refnum<vi>)
          n131 = Equal?(x=lveventtype."Key Repeat", y=w489) -> (x = y?=w487:bool)
          n132 = Equal?(x=lveventtype."Key Repeat?", y=w489) -> (x = y?=w488:bool)
          n133 = Or(x=w487, y=w488) -> (x .or. y?=w486:bool)
          n134 = case shown="\"Default\", Default" w483 {
            tunnel: w498 -> [_ w572 w666]
            tunnel: w497 -> [w503 w571 w669]
            tunnel: w496 -> [w505 w570 w674]
            tunnel: [w502 w569 w673] -> w495
            tunnel: [w501 w568 w668] -> w494
            tunnel: w493 -> [_ w567 _]
            tunnel: w492 -> [_ w566 _]
            tunnel: w485 -> [_ w565 w671]
            tunnel: w484 -> [_ w564 w667]
            tunnel: w482 -> [w504 w562 w672]
            tunnel: [w500 w561 w670] -> w480
            tunnel: w479 -> [w499 w560 _]
            tunnel: w478 -> [_ w559 _]
            frame "Default", Default {
              n135 = case shown="\"X\", \"x\"" w504 {
                tunnel: w505 -> [w514 w541 w548 w557]
                tunnel: w503 -> [w513 w540 w550 w558]
                tunnel: [w511 w541 w542 w552] -> w502
                tunnel: [w508 w540 w549 w553] -> w501
                tunnel: [w512 _ w546 w555] -> w500
                tunnel: w499 -> [w506 _ _ _]
                frame "V", "v" {
                  # "Paste"
                  n136 = call "NIIE_Read from Clipboard.vi"("Error"=w513, "Data"=w514) -> ("Error Out"=w509:errorcluster, "Key Focus Out"=w512:bool, "Data Out"=w510:T2, "Empty Clipboard String? Out"=w507:bool)  [unwired: 6 in]
                  n137 = case shown="True" w507 {
                    tunnel: [w517 w524] -> w511
                    tunnel: w510 -> [w516 w525]
                    tunnel: w509 -> [w515 w527]
                    tunnel: [w515 w521] -> w508
                    tunnel: w506 -> [_ w520]
                    frame False {
                      w519 = u32 111  # Invalid tool value
                      w518 = FALSE ("Support.CTRL Pressed")
                      n138 = Bundle By Name(cluster=w516, "Support.Shift pressed?"=w518, "Support.CTRL Pressed"=w518, "Support.Tool (old value)"=w519) -> (w517:T2)
                    }
                    frame True {
                      n139 = call "Empty Picture"() -> ("empty picture"=w528:picture)
                      n140 = call "Image_Get From Clipboard.vi"("Error"=w527, "Picture"=w528) -> ("Error Out"=w523:errorcluster, "Valid? Out"=w526:bool, "Picture Out"=w522:picture)  [unwired: 1 in, 6 out]
                      n141 = case shown="True" w526 {
                        tunnel: w525 -> [w530 w537]
                        tunnel: [w530 w533] -> w524
                        tunnel: w523 -> [w529 w538]
                        tunnel: w522 -> [_ w539]
                        tunnel: [w529 w532] -> w521
                        tunnel: w520 -> [_ w531]
                        frame False {
                        }
                        frame True {
                          n142 = call "NIIE_Create new layer_LayerName_Picture.vi"("Error"=w538, "Layer Name"=w531, "Picture"=w539, "Data"=w537) -> ("Error Out"=w536:errorcluster, "Data Out"=w535:T2)  [unwired: 6 in]
                          n143 = call "NIIE_Layer_View.vi"("Add To Undo?"=TRUE ("Add to Undo?"), "Error"=w536, "Data"=w535) -> ("Error Out"=w532:errorcluster, "Data Out"=w533:T2)  [unwired: 1 in, 6 out]
                        }
                      }
                    }
                  }
                }
                frame Default {
                }
                frame "C", "c" {
                  w545 = u32 111  # Invalid tool value
                  w544 = FALSE ("Support.CTRL Pressed")
                  n144 = call "NIIE_Write to Clipboard.vi"("Is Cut?"=FALSE, "Error"=w550, "Data"=w548) -> ("Error Out"=w549:errorcluster, "Key Focus Out"=w546:bool, "Data Out"=w543:T2)  [unwired: 6 in]
                  n145 = Bundle By Name(cluster=w543, "Support.Shift pressed?"=w544, "Support.CTRL Pressed"=w544, "Support.Tool (old value)"=w545) -> (w542:T2)
                }
                frame "X", "x" {
                  n146 = call "NIIE_Write to Clipboard.vi"("Is Cut?"=TRUE, "Error"=w558, "Data"=w557) -> ("Error Out"=w554:errorcluster, "Key Focus Out"=w555:bool, "Data Out"=w552:T2)  [unwired: 6 in]
                  n147 = Unbundle By Name(w552) -> ("Ref.Body Text"=w551:refnum<vi>)
                  n148 = call "NIIE_Fire Body Text Change event.vi"("error in"=w554, "Ref.Body Text"=w551) -> ("error out"=w553:errorcluster)  [unwired: 9 in]
                }
              }
            }
            frame "Tool" {
              n149 = Compound Arithmetic op=AND(invert w566, w567) -> (w563:bool)
              n150 = case shown="\"V\", \"v\"" w562 {
                tunnel: w572 -> [w585 _ _ _]
                tunnel: w571 -> [w584 w637 w655 w664]
                tunnel: w570 -> [w581 w641 w657 w665]
                tunnel: [w580 w639 w656 w659] -> w569
                tunnel: [w578 w640 w654 w661] -> w568
                tunnel: w563 -> [w577 _ _ _]
                tunnel: w565 -> [w576 _ _ _]
                tunnel: w564 -> [w575 _ _ _]
                tunnel: [_ w636 w652 w660] -> w561
                tunnel: w560 -> [_ w638 _ _]
                tunnel: w559 -> [w574 _ _ _]
                frame Default {
                  n151 = call "NIIE_IsAntsRectValid.vi"("Image Range"=w574) -> ("Valid? Out"=w573:bool)  [unwired: 10 out]
                  n152 = property class="RadioBtnsControl (strict)"(reference=w585, error in=w584) -> (reference out=w579:refnum<vi>, error out=w582:errorcluster, "Value"=w583:T12)
                  n153 = case shown="\"Select\"" w583 {
                    selector: w583 -> [w592 w611 _]
                    tunnel: w582 -> [w590 w614 w634]
                    tunnel: w581 -> [w594 w616 w635]
                    tunnel: [w593 w615 w633] -> w580
                    tunnel: w577 -> [w591 _ _]
                    tunnel: w579 -> [w589 w612 _]
                    tunnel: [w588 w613 w634] -> w578
                    tunnel: w576 -> [w587 w610 w632]
                    tunnel: w575 -> [w586 w609 w631]
                    tunnel: w573 -> [_ w617 _]
                    frame "Pencil", Default {
                      n154 = case shown="False" w591 {
                        tunnel: w594 -> [w599 w603]
                        tunnel: [w597 w608] -> w593
                        tunnel: w592 -> [_ w607]
                        tunnel: w590 -> [w598 w602]
                        tunnel: w589 -> [_ w606]
                        tunnel: [w598 w605] -> w588
                        tunnel: w587 -> [_ w601]
                        tunnel: w586 -> [_ w600]
                        frame False {
                          w596 = u32 111  # Invalid tool value
                          w595 = FALSE ("Support.CTRL Pressed")
                          n155 = Bundle By Name(cluster=w599, "Support.Shift pressed?"=w595, "Support.CTRL Pressed"=w595, "Support.Tool (old value)"=w596) -> (w597:T2)
                        }
                        frame True {
                          n156 = property class="RadioBtnsControl (strict)"(reference=w606, error in=w602, "Val(Sgnl)"=T12."Dropper" ("Value (Signaling)")) -> (error out=w605:errorcluster)  [unwired: 1 out]
                          n157 = Bundle By Name(cluster=w603, "Support.Tool (old value)"=w607, "Support.Shift pressed?"=w601, "Support.CTRL Pressed"=w600) -> (w608:T2)
                        }
                      }
                    }
                    frame "Select" {
                      n158 = case shown="True" w617 {
                        tunnel: w616 -> [w622 w630]
                        tunnel: [w621 w628] -> w615
                        tunnel: w614 -> [w625 w629]
                        tunnel: [w624 w629] -> w613
                        tunnel: w612 -> [w623 _]
                        tunnel: w611 -> [w620 _]
                        tunnel: w610 -> [w619 _]
                        tunnel: w609 -> [w618 _]
                        frame False {
                          n159 = Bundle By Name(cluster=w622, "Support.Tool (old value)"=w620, "Support.Shift pressed?"=w619, "Support.CTRL Pressed"=w618) -> (w621:T2)
                          n160 = property class="RadioBtnsControl (strict)"(reference=w623, error in=w625, "Val(Sgnl)"=T12."Dropper" ("Value (Signaling)")) -> (error out=w624:errorcluster)  [unwired: 1 out]
                        }
                        frame True {
                          w627 = u32 111  # Invalid tool value
                          n161 = Bundle By Name(cluster=w630, "Support.Tool (old value)"=w627) -> (w628:T2)
                        }
                      }
                    }
                    frame "Dropper" {
                      n162 = Bundle By Name(cluster=w635, "Support.Shift pressed?"=w632, "Support.CTRL Pressed"=w631) -> (w633:T2)
                    }
                  }
                }
                frame "V", "v" {
                  n163 = call "NIIE_Read from Clipboard.vi"("Error"=w637, "Data"=w641) -> ("Error Out"=w643:errorcluster, "Key Focus Out"=w636:bool, "Data Out"=w644:T2, "Empty Clipboard String? Out"=w642:bool)  [unwired: 6 in]
                  n164 = case shown="False" w642 {
                    tunnel: [w647 w650] -> w639
                    tunnel: w644 -> [w646 w650]
                    tunnel: w643 -> [w645 w651]
                    tunnel: [w645 w651] -> w640
                    tunnel: w638 -> [_ _]
                    frame False {
                      w649 = u32 111  # Invalid tool value
                      w648 = FALSE ("Support.CTRL Pressed")
                      n165 = Bundle By Name(cluster=w646, "Support.Shift pressed?"=w648, "Support.CTRL Pressed"=w648, "Support.Tool (old value)"=w649) -> (w647:T2)
                    }
                    frame True {
                    }
                  }
                }
                frame "C", "c" {
                  n166 = call "NIIE_Write to Clipboard.vi"("Is Cut?"=FALSE, "Error"=w655, "Data"=w657) -> ("Error Out"=w654:errorcluster, "Key Focus Out"=w652:bool, "Data Out"=w656:T2)  [unwired: 6 in]
                }
                frame "X", "x" {
                  n167 = call "NIIE_Write to Clipboard.vi"("Is Cut?"=TRUE, "Error"=w664, "Data"=w665) -> ("Error Out"=w662:errorcluster, "Key Focus Out"=w660:bool, "Data Out"=w659:T2)  [unwired: 6 in]
                  n168 = Unbundle By Name(w659) -> ("Ref.Body Text"=w658:refnum<vi>)
                  n169 = call "NIIE_Fire Body Text Change event.vi"("error in"=w662, "Ref.Body Text"=w658) -> ("error out"=w661:errorcluster)  [unwired: 9 in]
                }
              }
            }
            frame "Move Selection" {
              n170 = case shown="\"Z\", \"z\"" w672 {
                tunnel: w669 -> [w675 w682 w694]
                tunnel: w674 -> [w676 w681 w695]
                tunnel: [w676 w680 w692] -> w673
                tunnel: w671 -> [_ w679 _]
                tunnel: [_ w678 _] -> w670
                tunnel: [w675 w677 w693] -> w668
                tunnel: w667 -> [_ _ _]
                tunnel: w666 -> [_ _ _]
                frame Default {
                }
                frame "Z", "z" {
                  n171 = case shown="False" w679 {
                    tunnel: w682 -> [w686 w689]
                    tunnel: w681 -> [w688 w691]
                    tunnel: [w687 w691] -> w680
                    tunnel: [TRUE TRUE] -> w678
                    tunnel: [w685 w689] -> w677
                    frame False {
                      n172 = call "NIIE_Escape.vi"("Reset Cursor (T)"=FALSE ("Reset cursor (T)"), "Error"=w686, "Data"=w688) -> ("Error Out"=w685:errorcluster, "Data Out"=w687:T2)  [unwired: 7 out]
                    }
                    frame True {
                    }
                  }
                }
                frame "V", "v" {
                  n173 = call "NIIE_Finalize Movement.vi"("Error"=w694, "Data"=w695) -> ("Error Out"=w693:errorcluster, "Data Out"=w692:T2)  [unwired: 2 in, 6 out]
                }
              }
            }
          }
          n174 = Or(x=w480, y=w486) -> (x .or. y?=w481:bool)
        }
      }
    }
    frame Error {
    }
  }
  "Error Out" <- w9
  "Discard? Out" <- w5
  "Data Out" <- w3
